vi "TestXYGraph_Flow_v_Current_Plot_Dbl_VIG.vi"(4 "Plot Index/Size":i32, 6 "Point index/size":i32, 7 "Operation":T1(ring)=enum."set data", 8 "error in":errorcluster, 9 "XY Point":cluster{"X":dbl, "Y":dbl}, 11 "XY Graph":cluster{cluster{"X":dbl, "Y":dbl}[]}[](array[cluster])) -> (0 "error out":errorcluster, 2 "Current Flow and Limits vs Current":cluster{"X":dbl, "Y":dbl}[](array[cluster]), 3 "XY Graph":cluster{cluster{"X":dbl, "Y":dbl}[]}[](array[cluster]))   [LabVIEW 2018]
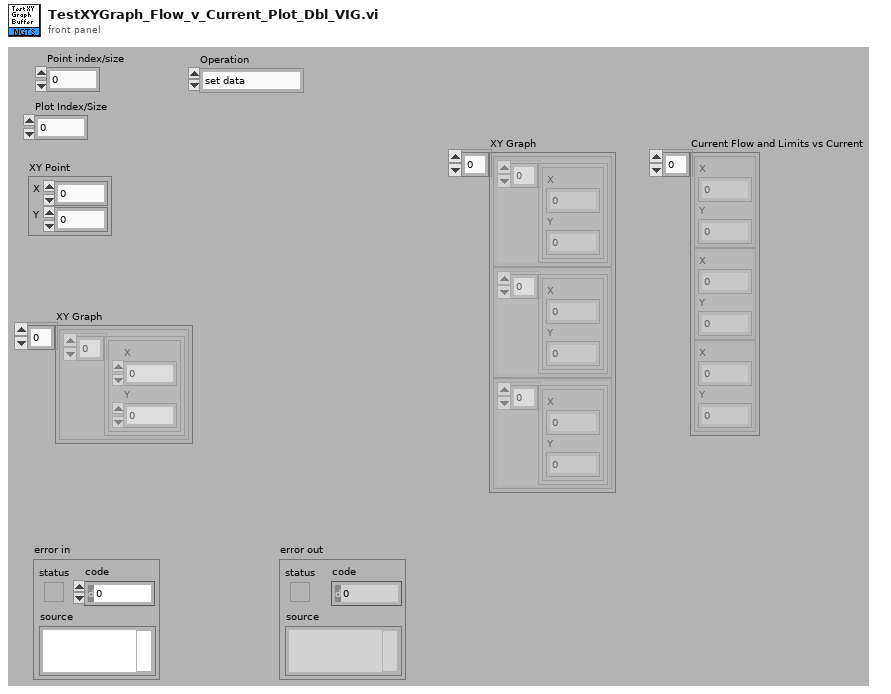
[diagram p1: front panel]
types:
  T1 = enum16{"get data", "set data", "Add Data Pair", "initialize"}
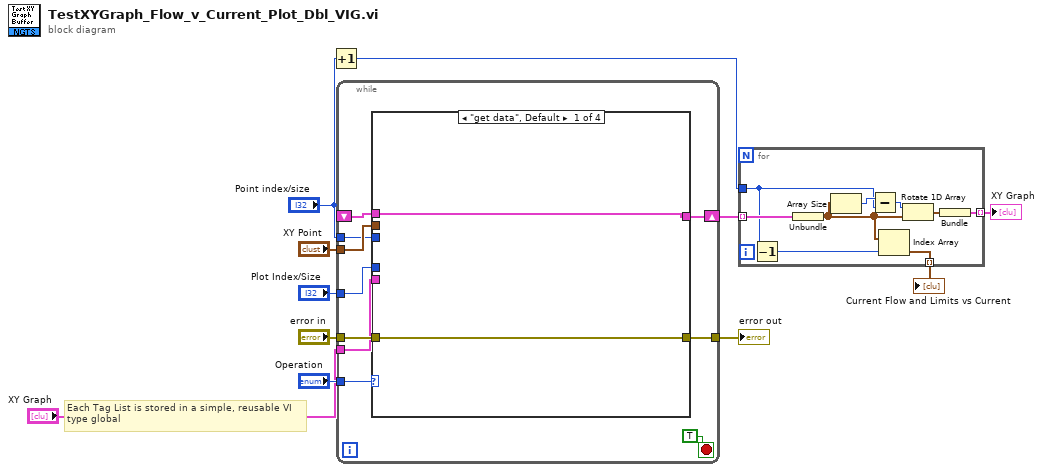
[diagram p0: block diagram]
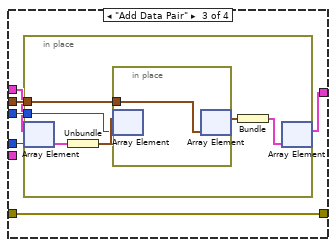
[diagram p3: hidden frame]
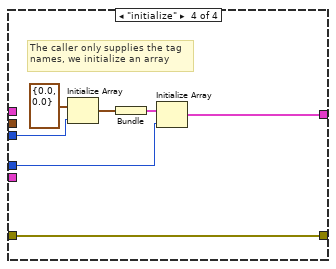
[diagram p4: hidden frame]
diagram:
  # "Each Tag List is stored in a simple, reusable VI\ntype global"
  n1 = Increment(x="Point index/size") -> (x+1=w3:i32)
  n2 = while {
    tunnel: "Operation" -> [w21]
    shift-right: [w19] -> w5
    shift-left: _ -> [w18]
    tunnel: "XY Point" -> [w17]
    tunnel: "error in" -> [w16]
    tunnel: [w15] -> w9
    tunnel: "Point index/size" -> [w14]
    tunnel: "Plot Index/Size" -> [w13]
    tunnel: "XY Graph" -> [w12]
    stop <- TRUE stop-if-true
    n3 = case shown="\"get data\", Default" w21 {
      tunnel: [w22 w24 w26 w39] -> w19
      tunnel: w18 -> [w22 _ w28 _]
      tunnel: w17 -> [_ _ w30 _]
      tunnel: w16 -> [w23 w25 w31 w45]
      tunnel: [w23 w25 w31 w45] -> w15
      tunnel: w14 -> [_ _ w29 w43]
      tunnel: w13 -> [_ _ w27 w40]
      tunnel: w12 -> [_ w24 _ _]
      frame "get data", Default {
      }
      frame "set data" {
      }
      frame "Add Data Pair" {
        n4 = in-place {
          in-place-border: w30 -> [w37]
          in-place-border: w29 -> [w32]
          n5 = in-place-array #1(w28, w27) -> (w35:cluster{cluster{"X":dbl, "Y":dbl}[]})
          n6 = Unbundle(w35) -> (w34:cluster{"X":dbl, "Y":dbl}[])
          n7 = in-place {
            in-place-border: w37 -> [w38]
            n8 = in-place-array #2(w34, w32) -> ()  [unwired: 1 out]
            n9 = in-place-array #2(w38) -> (w33:cluster{"X":dbl, "Y":dbl}[])  [unwired: 1 out]
          }
          n10 = Bundle(w33) -> (w36:cluster{cluster{"X":dbl, "Y":dbl}[]})  [unwired: 1 in]
          n11 = in-place-array #1(w36) -> (w26:cluster{cluster{"X":dbl, "Y":dbl}[]}[])  [unwired: 1 out]
        }
      }
      frame "initialize" {
        # "The caller only supplies the tag\nnames, we initialize an array"
        n12 = Initialize Array(cluster{"X":dbl, "Y":dbl} {"X"=0.0, "Y"=0.0} ("XYCluster"), w43) -> (w42:cluster{"X":dbl, "Y":dbl}[])
        n13 = Bundle(w42) -> (w41:cluster{cluster{"X":dbl, "Y":dbl}[]})  [unwired: 1 in]
        n14 = Initialize Array(w41, w40) -> (w39:cluster{cluster{"X":dbl, "Y":dbl}[]}[])
      }
    }
  }
  "error out" <- w9
  n15 = for {
    tunnel: w5 -> [w54] mode=indexing
    tunnel: [w52] -> w2 mode=indexing
    tunnel: w3 -> [w49]
    tunnel: [w47] -> w1 mode=indexing
    n16 = Decrement(x=w49) -> (x-1=w46:i32)
    n17 = Unbundle(w54) -> (w48:cluster{"X":dbl, "Y":dbl}[])
    n18 = Array Size(array=w48) -> (size(s)=w51:i32)
    n19 = Subtract(x=w51, y=w49) -> (x-y=w50:i32)
    n20 = Index Array(array=w48, index=w46) -> (element=w47:cluster{"X":dbl, "Y":dbl})
    n21 = Rotate 1D Array(1:w48, 2:w50) -> (0:w53:cluster{"X":dbl, "Y":dbl}[])
    n22 = Bundle(w53) -> (w52:cluster{cluster{"X":dbl, "Y":dbl}[]})  [unwired: 1 in]
  }
  "XY Graph" <- w2
  "Current Flow and Limits vs Current" <- w1
